vi "ARI Auto.vi"   [LabVIEW 2014]
uses:
  <vilib>/Platform/TimedLoop/XDataNode/timing_clust.ctl
  <vilib>/Platform/TimedLoop/XDataNode/nitl_modes.ctl
  <vilib>/Platform/TimedLoop/XDataNode/wakeup.ctl
  <vilib>/Rock Robotics/WPI/Relay/WPI_RelayValue.ctl
  <vilib>/platform/TimedLoop/XDataNode/XDataNode.xnode
  <vilib>/Platform/TimedLoop/XDataNode/XDNodeRunTimeDep.lvlib
types:
  T1 = typedef "XDNodeRunTimeDep.lvlib/timing_clust.ctl" = cluster{"Expected End [f-1]":u64, "Actual End [f-1]":u64, "Finished Late? [f-1]":bool, "Expected End [i-1]":u64, "Actual End [i-1]":u64, "Finished Late? [i-1]":bool, "Expected Start [i]":u64, "Actual Start [i]":u64, "Expected Start [f]":u64, "Actual Start [f]":u64, "Source Name":string, "Structure Name":string, "Period":i64, "Deadline":i64, "Offset":i64, "Start":i64, "Priority":i32, "Timeout":i32, "Mode":T2, "Wakeup Reason":T3, "Error":errorcluster, "Source Type":string, "Secondary Source Type":string, "Global End Time":u64, "Global Start Time":u64, "Frame Duration":u64, "Iteration Duration":u64, "Assigned CPU":i32, "I/O Scan Engine Mode":u32}
  T2 = typedef "XDNodeRunTimeDep.lvlib/nitl_modes.ctl" = enum32{"No Change", "Process missed periods, maintain original phase", "Discard missed periods, maintain original phase", "Process missed periods, ignore original phase", "Discard missed periods, ignore original phase"}
  T3 = typedef "XDNodeRunTimeDep.lvlib/wakeup.ctl" = enum32{"Normal", "Aborted", "Asynchronous wakeup", "Timing source error", "Timed loop error", "Timeout"}
  T4 = typedef "WPI_RelayValue.ctl" = enum16{"Off", "On", "Forward", "Reverse"}
  T5 = typedef "WPI_MotorControlDeviceRef.ctl" = cluster{"DeviceStatus":errorcluster, "Type":T6, "PWM":cluster{"Controller":T7, "PWM Channel":T8, "DeadBand":T9}, "CAN":cluster{"Device Number":u8, "Control Mode":T10, "Semaphore":T11, "Max Vout":dbl, "TalonSRX Control Mode":T12}, "Invert":bool, "TransformRef":T13, "InvTransformRef":T13}
  T6 = typedef "WPI_MotorControlType.ctl" = enum16{"PWM", "CAN", "CANTalonSRX"}
  T7 = typedef "FPGA_TypedefDigitalModule.ctl" = enum16{"Controller 1"}
  T8 = typedef "FPGA_DIOPWMChannel.ctl" = enum8{"PWM 0", "PWM 1", "PWM 2", "PWM 3", "PWM 4", "PWM 5", "PWM 6", "PWM 7", "PWM 8", "PWM 9", "PWM MXP 0", "PWM MXP 1", "PWM MXP 2", "PWM MXP 3", "PWM MXP 4", "PWM MXP 5", "PWM MXP 6", "PWM MXP 7", "PWM MXP 8", "PWM MXP 9", "Invalid"}
  T9 = typedef "WPI_PWMDeadband.ctl" = cluster{"Name":string, "maxPositivePwm":i32, "minPositivePwm":i32, "centerPwm":i32, "maxNegativePwm":i32, "minNegativePwm":i32, "angularRange":u16}
  T10 = typedef "WPI_CANJaguar_ControlMode.ctl" = enum8{"Percent VBus", "Current", "Speed", "Position", "Voltage"}
  T11 = typedef "Semaphore RefNum" = refnum<k1>
  T12 = typedef "WPI_CANTalonSRX_APIControlMode.ctl" = enum8{"Percent VBus", "Speed", "Position", "Slave", "Unchanged / Invalid"}
  T13 = typedef "WPI_PWMTransform_ConPane.ctl" = refnum<vi>
  T14 = typedef "WPI_RelayDevRef.ctl" = cluster{"DevStatus":errorcluster, "Relay Channel":T15, "Controller":T7, "Relay Direction":T16}
  T15 = typedef "FPGA_DIORelayChannel.ctl" = enum8{"Relay 0", "Relay 1", "Relay 2", "Relay 3", "Invalid"}
  T16 = typedef "WPI_RelayDirection.ctl" = enum16{"Both directions", "Forward only", "Reverse only"}
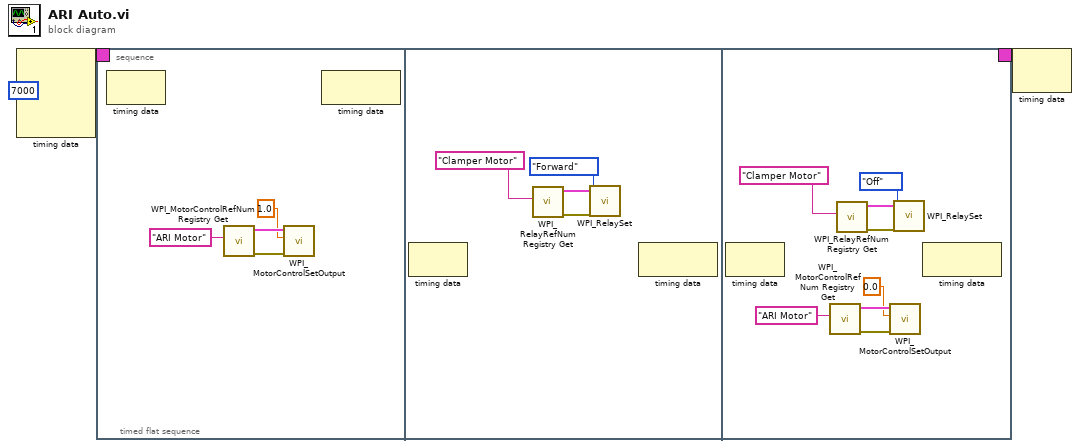
[diagram p0: block diagram]
diagram:
  n1 = node-c288(i64 7000 ("Offset")) -> (w3:T1)  [unwired: 3 in]
  n2 = timed-sequence {
    timing: w3 -> [_]
    timing-out: [_] -> w2
    n3 = timed-flat-sequence {
      frame #0 {
        n4 = node-c288() -> ()  [unwired: 1 in, 1 out]
        n5 = call <vilib>:"WPI_MotorControlRefNum Registry Get.vi"("refnum name"="ARI Motor") -> ("error out"=w7:errorcluster, "MotorControlDevRef"=w6:T5)  [unwired: 9 in]
        n6 = call <vilib>:"WPI_MotorControlSetOutput.vi"("error in (no error)"=w7, "Output"=1.0, "MotorControlDevRef"=w6) -> ()  [unwired: 6 in, 3 out]
        n7 = node-c288() -> ()  [unwired: 1 in, 1 out]
      }
      frame #1 {
        n8 = node-c288() -> ()  [unwired: 1 in, 1 out]
        n9 = call <vilib>:"WPI_RelayRefNum Registry Get.vi"("refnum name"="Clamper Motor") -> ("error out"=w12:errorcluster, "RelayDevRef"=w13:T14)  [unwired: 9 in]
        n10 = call <vilib>:"WPI_RelaySet.vi"("error in (no error)"=w12, "RelayValue"=WPI_RelayValue."Forward", "RelayDevRef"=w13) -> ()  [unwired: 7 in, 2 out]
        n11 = node-c288() -> ()  [unwired: 1 in, 1 out]
      }
      frame #2 {
        n12 = node-c288() -> ()  [unwired: 1 in, 1 out]
        n13 = call <vilib>:"WPI_MotorControlRefNum Registry Get.vi"("refnum name"="ARI Motor") -> ("error out"=w19:errorcluster, "MotorControlDevRef"=w18:T5)  [unwired: 9 in]
        n14 = call <vilib>:"WPI_RelayRefNum Registry Get.vi"("refnum name"="Clamper Motor") -> ("error out"=w22:errorcluster, "RelayDevRef"=w23:T14)  [unwired: 9 in]
        n15 = call <vilib>:"WPI_MotorControlSetOutput.vi"("error in (no error)"=w19, "Output"=0.0, "MotorControlDevRef"=w18) -> ()  [unwired: 6 in, 3 out]
        n16 = call <vilib>:"WPI_RelaySet.vi"("error in (no error)"=w22, "RelayValue"=WPI_RelayValue."Off", "RelayDevRef"=w23) -> ()  [unwired: 7 in, 2 out]
        n17 = node-c288() -> ()  [unwired: 1 in, 1 out]
      }
    }
  }
  n18 = node-c288(w2) -> ()  [unwired: 1 out]
